vi "最小窗口后台运行(子VI).vi"(10 "App.Kind":T1(ring), 11 "停止输入":bool caption="停止 2") -> (0 "错误输出":errorcluster)   [LabVIEW 2016, in "数据传输系统-02.lvlib"]
uses:
  <vilib>/Averna/Notify Icon/NotifyIcon.llb/BalloonIcon.ctl
  <vilib>/Averna/Notify Icon/NotifyIcon.llb/GetSelectedItemEvent.vi
  <vilib>/Averna/Notify Icon/NotifyIcon.llb/SetVisible.vi
  <vilib>/Averna/Notify Icon/NotifyIcon.llb/SetMenuDefaultItem.vi
  <vilib>/Averna/Notify Icon/NotifyIcon.llb/SetTipText.vi
  <vilib>/Averna/Notify Icon/NotifyIcon.llb/NotifyIcon.lvclass
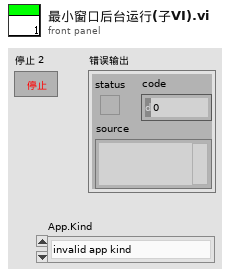
[diagram p1: front panel]
types:
  T1 = enum32{"invalid app kind", "Development System", "Run Time System", "Student Edition", "Embedded LabVIEW", "Evaluation", "Custom"}
  T2 = enum32{"Invalid", "Standard", "Closed", "Hidden", "Minimized", "Maximized"}
  T3 = typedef "NotifyIcon.lvlib/NotifyIcon.lvclass/BalloonIcon.ctl" = enum32{"None", "Information", "Warning", "Error"}
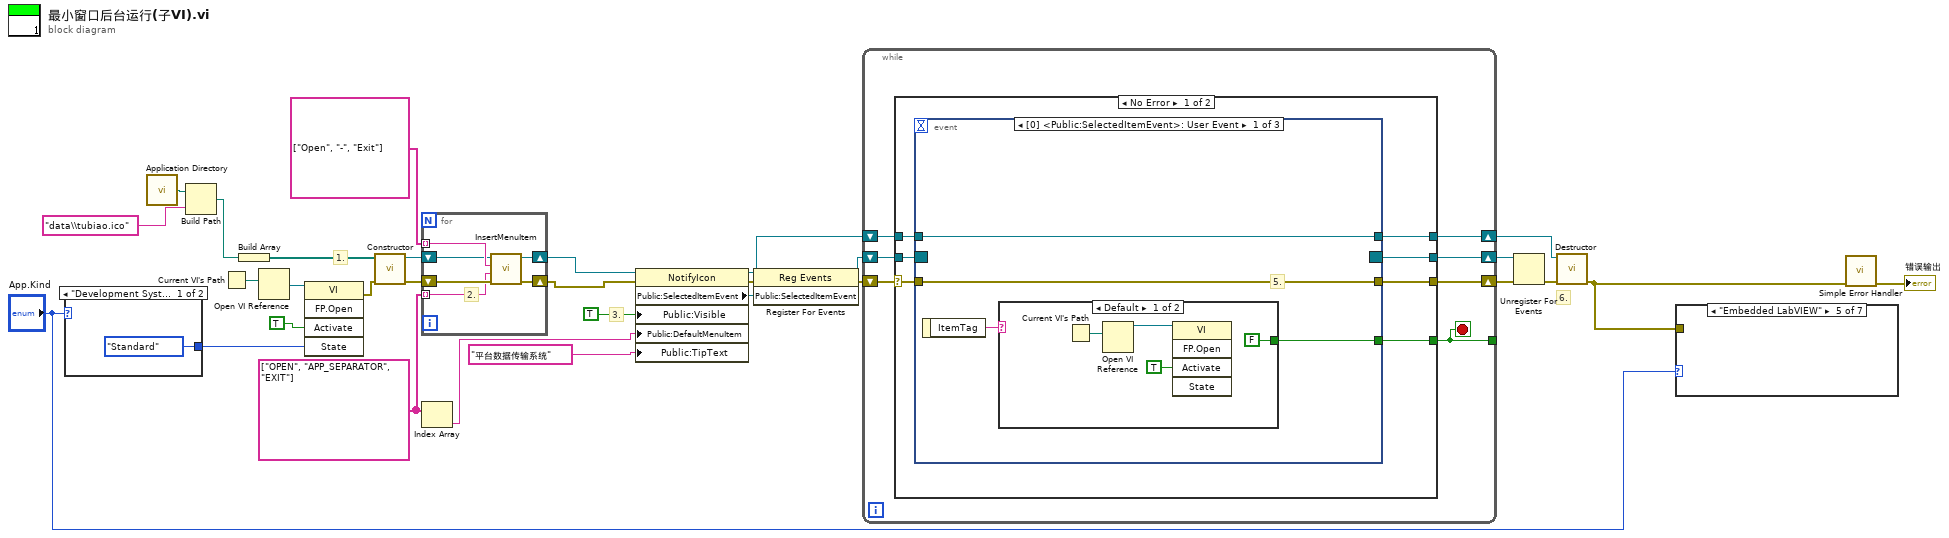
[diagram p0: block diagram]
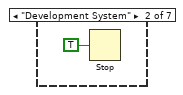
[diagram p3: hidden frame]
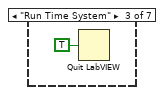
[diagram p4: hidden frame]
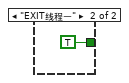
[diagram p8: hidden frame]
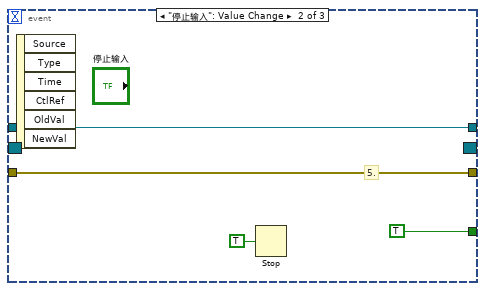
[diagram p9: hidden frame]
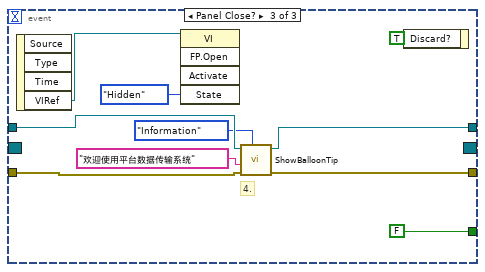
[diagram p10: hidden frame]
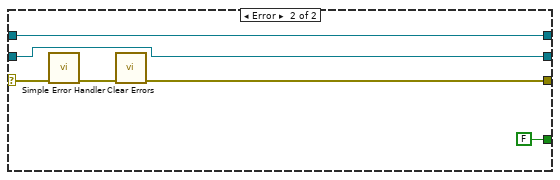
[diagram p11: hidden frame]
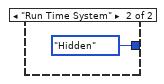
[diagram p12: hidden frame]
diagram:
  w9 = string[] ["OPEN", "APP_SEPARATOR", "EXIT"]
  # "6."
  # "3."
  # "1."
  n1 = case shown="\"Development System\", Default" "App.Kind" {
    tunnel: [T2."Standard" ("状态") T2."Hidden" ("状态")] -> w28
    frame "Development System", Default {
    }
    frame "Run Time System" {
    }
  }
  n2 = call <vilib>:"Application Directory.vi"() -> ("Application Directory"=w7:path)
  n3 = Build Path(base path=w7, name or relative path="data\\tubiao.ico" ("名称或相对路径")) -> (appended path=w17:path)
  n4 = Current VI's Path() -> (path=w4:path)
  n5 = Build Array(w17) -> (w12:path[])
  n6 = Open VI Reference(vi path=w4) -> (vi reference=w3:refnum<vi>)  [unwired: 5 in, 1 out]
  n7 = invoke class="VI" method="FP.Open"(reference=w3, "Activate"=TRUE ("激活？"), "State"=w28) -> (error out=w2:errorcluster)  [unwired: 2 in, 4 out]
  n8 = call <vilib>:"Constructor.vi"("error in"=w2, "IconFilePathList"=w12) -> ("error out"=w16:errorcluster, "NotifyIcon"=w8:refnum<class "NotifyIcon.lvclass">)  [unwired: 8 in]
  n9 = for {
    shift-right: [w37] -> w30
    shift-left: w16 -> [w38]
    tunnel: string[] ["Open", "-", "Exit"] -> [w36] mode=indexing
    tunnel: w9 -> [w35] mode=indexing
    shift-right: [w33] -> w29
    shift-left: w8 -> [w34]
    # "2."
    n10 = call <vilib>:"InsertMenuItem.vi"("error in"=w38, "ItemTag"=w35, "ItemName"=w36, "NotifyIcon in"=w34) -> ("error out"=w37:errorcluster, "NotifyIcon out"=w33:refnum<class "NotifyIcon.lvclass">)  [unwired: 6 in]
  }
  n11 = Index Array(array=w9) -> (element=w10:string)  [unwired: 1 in]
  n12 = property class="NotifyIcon"(reference=w29, error in=w30, "Public:Visible"=TRUE ("Visible"), "Public:DefaultMenuItem"=w10, "Public:TipText"="平台数据传输系统" ("TipText")) -> (reference out=w24:refnum<class "NotifyIcon.lvclass">, error out=w15:errorcluster, "Public:SelectedItemEvent"=w14:refnum<user-event>)
  n13 = register-events(error in=w15, w14) -> (reference out=w25:refnum<event-registration>, error out=w26:errorcluster)  [unwired: 1 in]
  n14 = while {
    shift-right: [w42] -> w22
    shift-left: w26 -> [w41]
    shift-right: [w43] -> w19
    shift-left: w24 -> [w44]
    shift-right: [w40] -> w20
    shift-left: w25 -> [w45]
    tunnel: [w39] -> _
    stop <- w39 stop-if-true
    n15 = case shown="No Error" w41 {
      selector: w41 -> [w47 w81]
      tunnel: w45 -> [w52 w76]
      tunnel: w44 -> [w51 w77]
      tunnel: [w50 w77] -> w43
      tunnel: [w49 w79] -> w42
      tunnel: [w48 FALSE ("Discard?")] -> w39
      tunnel: [w46 w76] -> w40
      frame No Error {
        n16 = event shown="[0] <Public:SelectedItemEvent>: User Event" {
          selector: w52 -> [_ _ _]
          dyn-events: [_ _ _] -> w46
          timeout: _ -> [_ _ _]
          tunnel: w47 -> [w55 w65 w74]
          tunnel: [w55 w65 w73] -> w49
          tunnel: [w54 TRUE FALSE ("Discard?")] -> w48
          tunnel: w51 -> [w53 w63 w75]
          tunnel: [w53 w63 w72] -> w50
          event User Event {
            # "5."
            n17 = event-data() -> ("ItemTag"=w56:string)  [unwired: 1 in]
            n18 = case shown="Default" w56 {
              tunnel: [FALSE TRUE] -> w54
              frame Default {
                n19 = Current VI's Path() -> (path=w57:path)
                n20 = Open VI Reference(vi path=w57) -> (vi reference=w58:refnum<vi>)  [unwired: 5 in, 1 out]
                n21 = invoke class="VI" method="FP.Open"(reference=w58, "Activate"=TRUE ("激活？")) -> ()  [unwired: 3 in, 5 out]
              }
              frame "EXIT线程一" {
              }
            }
          }
          event "停止输入": Value Change {
            # "5."
            n22 = event-data() -> ()  [unwired: 1 in, 6 out]
            n23 = Stop(stop? (T)=TRUE ("可见")) -> ()
          }
          event Panel Close? {
            # "4."
            n24 = event-data() -> ("VIRef"=w68:refnum<vi>)  [unwired: 1 in, 3 out]
            n25 = invoke class="VI" method="FP.Open"(reference=w68, "State"=T2."Hidden" ("状态")) -> ()  [unwired: 3 in, 5 out]
            n26 = call <vilib>:"ShowBalloonTip.vi"("Balloon Icon"=BalloonIcon."Information", "error in"=w74, "Text"="欢迎使用平台数据传输系统", "NotifyIcon in"=w75) -> ("error out"=w73:errorcluster, "NotifyIcon out"=w72:refnum<class "NotifyIcon.lvclass">)  [unwired: 6 in]
            n27 = event-data("Discard?"=TRUE ("放弃？")) -> ()  [unwired: 1 in, 1 out]
          }
        }
      }
      frame Error {
        n28 = call <vilib>:"Simple Error Handler.vi"("error in (no error)"=w81) -> ("error out"=w80:errorcluster)  [unwired: 4 in, 4 out]
        n29 = call <vilib>:"Clear Errors.vi"("error in (no error)"=w80) -> ("error out"=w79:errorcluster)  [unwired: 5 in, 1 out]
      }
    }
  }
  n30 = Unregister For Events(event registration refnum=w20, error in=w22) -> (error out=w23:errorcluster)
  n31 = call <vilib>:"Destructor.vi"("error in"=w23, "NotifyIcon"=w19) -> ("error out"=w18:errorcluster)  [unwired: 9 in]
  n32 = case shown="\"Embedded LabVIEW\"" "App.Kind" {
    tunnel: w18 -> [_ _ _ _ _ _ _]
    frame "invalid app kind", Default {
    }
    frame "Development System" {
      n33 = Stop(stop? (T)=TRUE ("可见")) -> ()
    }
    frame "Run Time System" {
      n34 = Quit LabVIEW(quit? (T)=TRUE ("退出？(T)")) -> ()
    }
    frame "Student Edition" {
    }
    frame "Embedded LabVIEW" {
    }
    frame "Evaluation" {
    }
    frame "Custom" {
    }
  }
  n35 = call <vilib>:"Simple Error Handler.vi"("error in (no error)"=w18) -> ("error out"=→"错误输出":errorcluster)  [unwired: 4 in, 4 out]
